vi "Get Register Data.vi"(8 "error in (no error)":errorcluster, 11 "RFFE Extended Command in":refnum<class "RFFE Extended Command.lvclass">) -> (0 "error out":errorcluster, 2 "Register Data":T1[](array[typedef]) format="%02x", 3 "RFFE Extended Command out":refnum<class "RFFE Extended Command.lvclass">)   [LabVIEW 2018, in "MIPI RFFE API.lvlib" / "RFFE Extended Command.lvclass"]
uses:
  RFFE Extended Command.lvclass
  Register Data.ctl
  RFFE Extended Command.lvclass/RFFE Extended Command.ctl
  MIPI RFFE API.lvlib
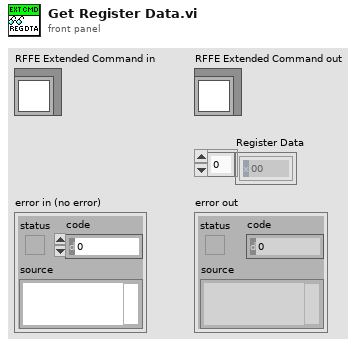
[diagram p1: front panel]
types:
  T1 = typedef "MIPI RFFE API.lvlib/Register Data.ctl" = u8
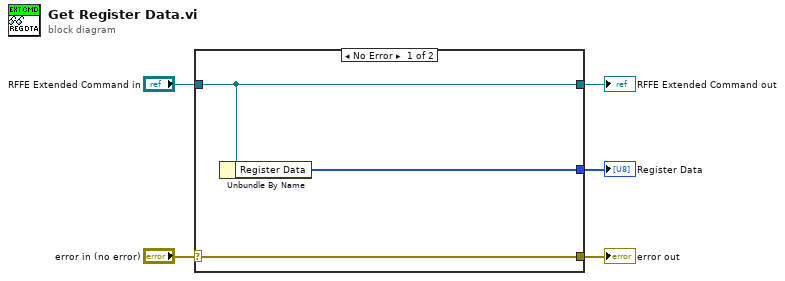
[diagram p0: block diagram]
diagram:
  n1 = case shown="No Error" "error in (no error)" {
    selector: "error in (no error)" -> [w8 w9]
    tunnel: [w8 w9] -> w4
    tunnel: [w7 w10] -> w2
    tunnel: "RFFE Extended Command in" -> [w7 w10]
    tunnel: [w6 _] -> w1
    frame No Error {
      n2 = Unbundle By Name(w7) -> ("Register Data"=w6:T1[])
    }
    frame Error {
    }
  }
  "error out" <- w4
  "RFFE Extended Command out" <- w2
  "Register Data" <- w1
